vi "Cleanup.vi"(7 "Msg":refnum<class "Msg.lvclass">) -> ()   [LabVIEW 2020, in "jettl.lvlib" / "Msg.lvclass"]
uses:
  Msg.lvclass
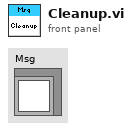
[diagram p1: front panel]
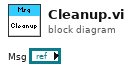
[diagram p0: block diagram]
diagram:
